vi "TLV Frame.vi"(8 "error in (no error)":errorcluster, 10 "TLV Frame":T1, 11 "Protocol Verification Test in":refnum<class "Protocol Verification Test.lvclass">) -> (0 "error out":errorcluster, 3 "Protocol Verification Test out":refnum<class "Protocol Verification Test.lvclass">)   [LabVIEW 2017, in "Protocol Verification Test.lvlib" / "Protocol Verification Test.lvclass"]
uses:
  Protocol Verification Test.lvclass
  TLV Data.ctl
  Protocol Verification Test.lvclass/Protocol Verification Test.ctl
  Protocol Verification Test.lvlib
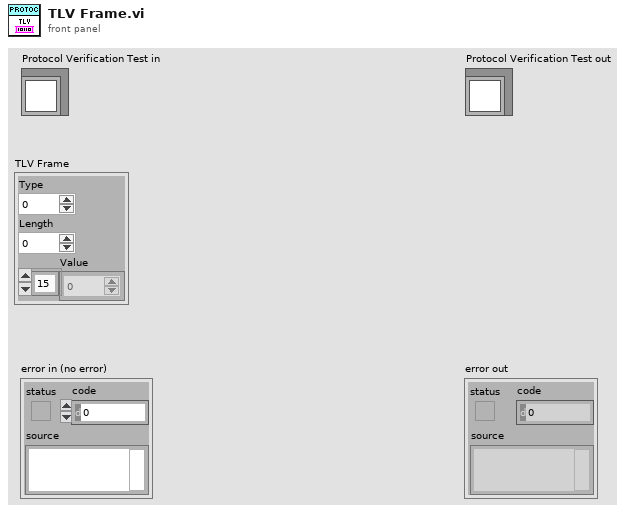
[diagram p1: front panel]
types:
  T1 = typedef "Protocol Verification Test.lvlib/TLV Data.ctl" = cluster{"Type":u8, "Length":u8, "Value":u8[]}
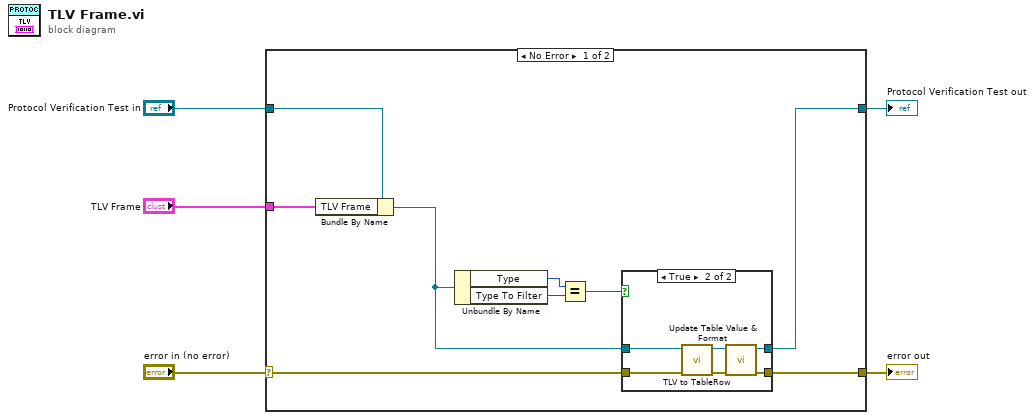
[diagram p0: block diagram]
diagram:
  n1 = case shown="No Error" "error in (no error)" {
    selector: "error in (no error)" -> [w12 w24]
    tunnel: [w11 w24] -> w4
    tunnel: [w10 w23] -> w2
    tunnel: "Protocol Verification Test in" -> [w14 w23]
    tunnel: "TLV Frame" -> [w13 _]
    frame No Error {
      n2 = Bundle By Name(cluster=w14, "TLV Frame"=w13) -> (w9:refnum<class "Protocol Verification Test.lvclass">)
      n3 = Unbundle By Name(w9) -> ("Type"=w8:u8, "Type To Filter"=w7:i32)
      n4 = Equal?(x=w8, y=w7) -> (x = y?=w6:bool)
      n5 = case shown="True" w6 {
        tunnel: w12 -> [w16 w22]
        tunnel: [w16 w19] -> w11
        tunnel: [w15 w18] -> w10
        tunnel: w9 -> [w15 w17]
        frame False {
        }
        frame True {
          n6 = call "TLV to TableRow.vi"("error in (no error)"=w22, "Protocol Verification Test in"=w17) -> ("error out"=w20:errorcluster, "Protocol Verification Test out"=w21:refnum<class "Protocol Verification Test.lvclass">)  [unwired: 8 in]
          n7 = call "Update Table Value & Format.vi"("error in (no error)"=w20, "Protocol Verification Test in"=w21) -> ("error out"=w19:errorcluster, "Protocol Verification Test out"=w18:refnum<class "Protocol Verification Test.lvclass">)  [unwired: 8 in]
        }
      }
    }
    frame Error {
    }
  }
  "error out" <- w4
  "Protocol Verification Test out" <- w2
